vi "HeadPan.vi"(0 "error in":errorcluster, 2 "Parameters":T1={"Pan Angle"=0.0, "Speed"=50, "Units"=enum."Degrees"}, 3 "node":string) -> (1 "error out":errorcluster)   [LabVIEW 2015]
doc: "This VI sets the head to pan to a given angle at a given speed"
uses:
  ROS/Code/Console/Servers/ServerSubs/TopicDef.ctl
  ROS/Code/SubVIs/_ROSDirection.ctl
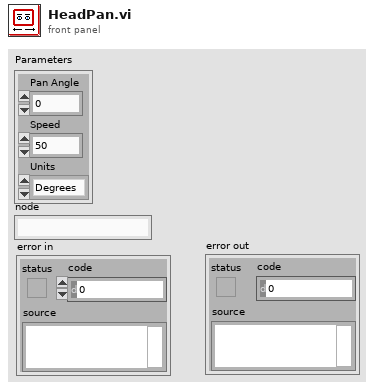
[diagram p1: front panel]
types:
  T1 = cluster{"Pan Angle":sgl, "Speed":i32, "Units":enum16{"Degrees", "Radians"}}
  T2 = typedef "TopicDef.ctl" = cluster{"Topic":string, "Type":string, "Action":T3, "Update (ms)":u16, "queue size":u16}
  T3 = typedef "_ROSDirection.ctl" = enum16{"Node", "Publisher", "Subscriber", "ServiceClient", "ServiceProvider"}
  T4 = typedef "_ROSControl.ctl" = cluster{"topic port":u16, "Node":string, "topic":string, "type":string, "node port":u16, "error ":errorcluster, "Direction":T3, "Update (ms)":u16, "FIFO size":u16}
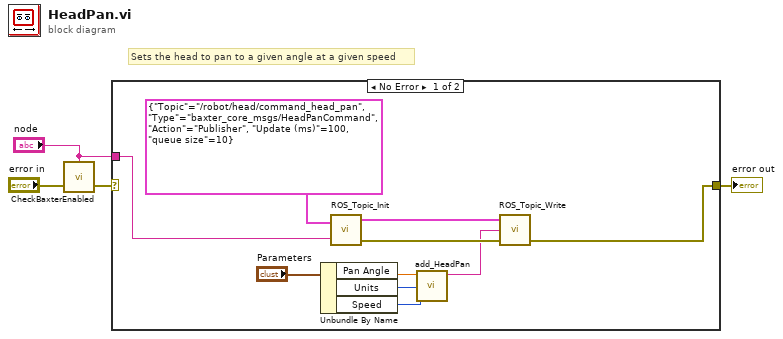
[diagram p0: block diagram]
diagram:
  # "Sets the head to pan to a given angle at a given speed"
  n1 = call "CheckBaxterEnabled.vi"("error in"="error in", "node"="node") -> ("error out"=w2:errorcluster)  [unwired: 2 in]
  n2 = case shown="No Error" w2 {
    selector: w2 -> [_ w15]
    tunnel: [w5 w15] -> w4
    tunnel: "node" -> [w12 _]
    frame No Error {
      n3 = Unbundle By Name("Parameters") -> ("Pan Angle"=w10:sgl, "Units"=w9:enum16{"Degrees", "Radians"}, "Speed"=w8:i32)
      n4 = call "ROS_Topic_Init.vi"("Definitions"=T2 {"Topic"="/robot/head/command_head_pan", "Type"="baxter_core_msgs/HeadPanCommand", "Action"=enum."Publisher", "Update (ms)"=100, "queue size"=10}, "node"=w12) -> ("ROS out"=w14:T4, "error out"=w7:errorcluster)  [unwired: 1 in]
      n5 = call "add_HeadPan.vi"("Speed"=w8, "Units"=w9, "Pan Angle"=w10) -> ("msg out"=w6:string)  [unwired: 8 in]
      n6 = call "ROS_Topic_Write.vi"("error in (no error)"=w7, "Msg in"=w6, "ROS in"=w14) -> ("error out"=w5:errorcluster)  [unwired: 1 in, 1 out]
    }
    frame Error {
    }
  }
  "error out" <- w4
